vi "Configure Data Marker [DM] Core.vi"(6 "Destination Terminal (None)":string(combo) caption="destination terminal (None)", 7 "Bit Position":i32 caption="bit position" format="%.0g", 8 "error in (no error)":errorcluster, 9 "Marker Name (\"\")":string caption="marker name (\"\")", 10 "Source Channel (\"\")":string="CHANNEL1" caption="source channel (\"CHANNEL1\")", 11 "IVI_Fgen in":refnum<class "IVI_Fgen.lvclass">) -> (0 "error out":errorcluster, 3 "IVI_Fgen out":refnum<class "IVI_Fgen.lvclass">)   [LabVIEW 2013, in "IVI_Fgen.lvlib" / "IVI_Fgen.lvclass"]
doc: "This VI configures the common data marker properties. These properties are the data marker source channel, bit position, and destination.\n \nNote:\n\n(1) This VI is part of the IviFgenDataMarker [DM] extension group."
uses:
  IVI_Fgen.lvclass
  IVI_Fgen.lvclass/IVI_Fgen.ctl
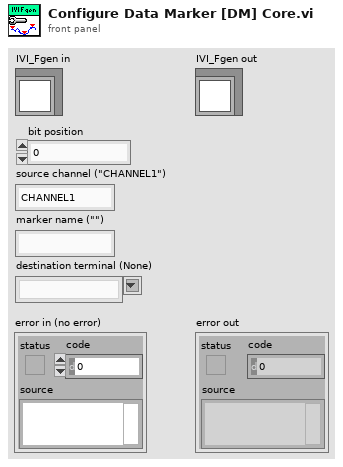
[diagram p1: front panel]
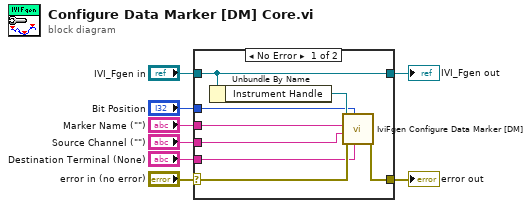
[diagram p0: block diagram]
diagram:
  n1 = case shown="No Error" "error in (no error)" {
    selector: "error in (no error)" -> [w14 w18]
    tunnel: [w13 w18] -> w7
    tunnel: [w16 w17] -> w5
    tunnel: "IVI_Fgen in" -> [w16 w17]
    tunnel: "Bit Position" -> [w12 _]
    tunnel: "Marker Name (\"\")" -> [w11 _]
    tunnel: "Source Channel (\"\")" -> [w10 _]
    tunnel: "Destination Terminal (None)" -> [w9 _]
    frame No Error {
      n2 = Unbundle By Name(w16) -> ("Instrument Handle"=w15:refnum<k15>)
      n3 = call <vilib>:"IviFgen Configure Data Marker [DM].vi"("Destination Terminal (None)"=w9, "Bit Position"=w12, "error in (no error)"=w14, "Source Channel (\"\")"=w10, "Marker Name (\"\")"=w11, "instrument handle"=w15) -> ("error out"=w13:errorcluster)  [unwired: 4 in, 1 out]
    }
    frame Error {
    }
  }
  "error out" <- w7
  "IVI_Fgen out" <- w5
